vi "GE5565 DMA Read Interrupt (U64) Cluster.vi"(6 "timeout (1000 ms)":u32=1000, 8 "error in (no error)":errorcluster, 10 "RM offset (0)":u32, 11 "VMIC reference in":T1) -> (0 "error out":errorcluster, 2 "buffer":dbl[](array[numeric]), 3 "VMIC reference out":T1)   [LabVIEW 2020, in "RefMem DMA Engine.lvlib"]
uses:
  RefMem DMA Engine.lvlib
  <vilib>/Instr/_visa.llb/Select Event Type.ctl
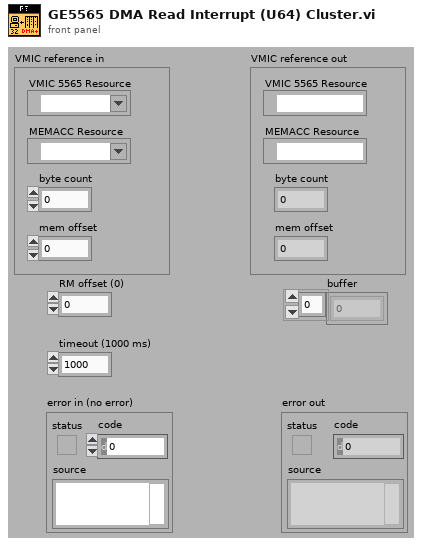
[diagram p1: front panel]
types:
  T1 = cluster{"VMIC 5565 Resource":refnum<visa-resource-name>, "MEMACC Resource":refnum<visa-resource-name>, "byte count":u32, "mem offset":u32}
  T2 = enum16{"big-endian, network order", "native, host order", "little-endian"}
  T3 = typedef "Select Event Type.ctl" = u32
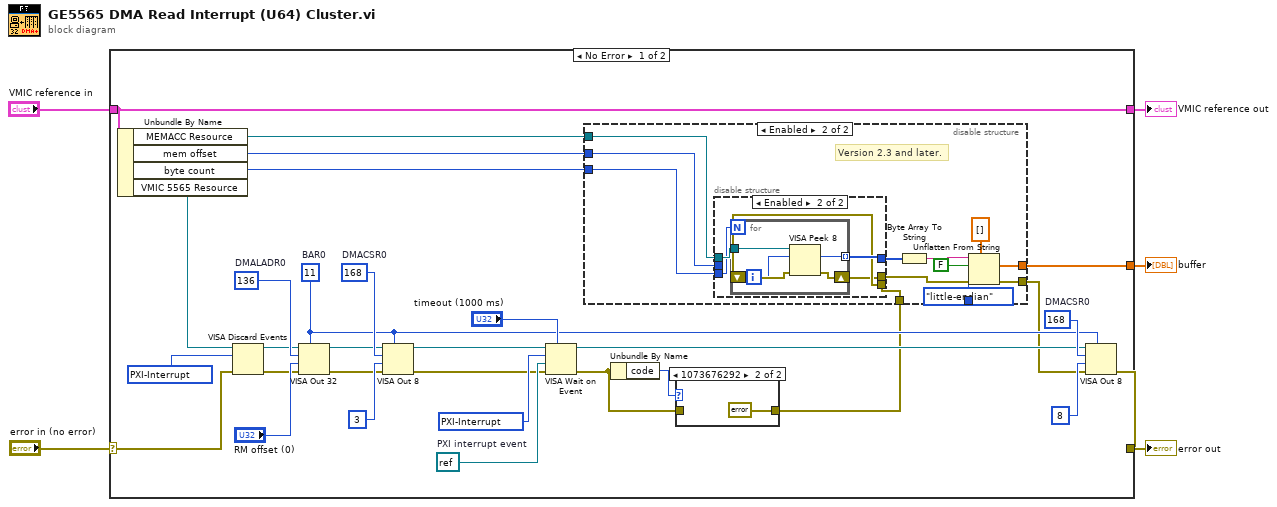
[diagram p0: block diagram]
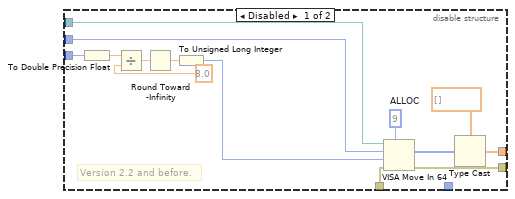
[diagram p2: hidden frame]
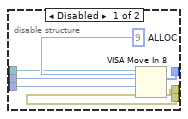
[diagram p3: hidden frame]
diagram:
  n1 = case shown="No Error" "error in (no error)" {
    selector: "error in (no error)" -> [w26 w82]
    tunnel: "VMIC reference in" -> [w21 w83]
    tunnel: [w21 w83] -> w2
    tunnel: [w11 w82] -> w4
    tunnel: [w10 _] -> w1
    frame No Error {
      w13 = u16 11  # BAR0
      w28 = refnum<visa-resource-name> refnum  # PXI interrupt event
      w16 = u32 168  # DMACSR0
      w23 = T3 1073684514 items=["ServiceRequest"=1073684491, "Trigger"=3221168138, "Clear"=1073684493, "VXI-Signal"=1073684512, "VXI/VME-Interrupt"=3221168161, "VXI/VME-Sysfail"=1073684509, "VXI/VME-Sysreset"=1073684510, "GPIB-CIC"=1073684498, "GPIB-Talk"=1073684499, "GPIB-Listen"=1073684500, "PXI-Interrupt"=1073684514, "AllEnabled"=1073709055] ("Event Type")
      w29 = T3 1073684514 items=["ServiceRequest"=1073684491, "Trigger"=3221168138, "Clear"=1073684493, "VXI-Signal"=1073684512, "VXI/VME-Interrupt"=3221168161, "VXI/VME-Sysfail"=1073684509, "VXI/VME-Sysreset"=1073684510, "GPIB-CIC"=1073684498, "GPIB-Talk"=1073684499, "GPIB-Listen"=1073684500, "PXI-Interrupt"=1073684514, "AllEnabled"=1073709055] ("Event Type")
      w35 = u32 168  # DMACSR0
      w36 = u32 136  # DMALADR0
      n2 = Unbundle By Name(w21) -> ("MEMACC Resource"=w18:refnum<visa-resource-name>, "mem offset"=w19:u32, "byte count"=w20:u32, "VMIC 5565 Resource"=w22:refnum<visa-resource-name>)
      n3 = VISA Discard Events(8:w26, 10:w23, 11:w22) -> (0:w24:errorcluster, 3:w25:refnum<visa-resource-name>)  [unwired: 1 in]
      n4 = VISA Out 32(7:w13, 8:w24, 9:"RM offset (0)", 10:w36, 11:w25) -> (0:w32:errorcluster, 3:w33:refnum<visa-resource-name>)
      n5 = VISA Out 8(7:w13, 8:w32, 9:u8 3 ("value (0)"), 10:w35, 11:w33) -> (0:w17:errorcluster, 3:w27:refnum<visa-resource-name>)
      n6 = VISA Wait on Event(7:"timeout (1000 ms)", 8:w17, 9:w28, 10:w29, 11:w27) -> (0:w9:errorcluster, 3:w14:refnum<visa-resource-name>)  [unwired: 2 out]
      n7 = Unbundle By Name(w9) -> ("code"=w7:i32)
      n8 = case shown="1073676292" w7 {
        tunnel: [w80 errorcluster {"status"=FALSE, "code"=0, "source"=""} ("error out")] -> w8
        tunnel: w9 -> [w80 _]
        frame 0, Default {
        }
        frame 1073676292 {
        }
      }
      n9 = disable-structure shown="Enabled" {
        disable-tunnel: w20 -> [w44 w52]
        disable-tunnel: w19 -> [w43 w53]
        disable-tunnel: w18 -> [w42 w54]
        disable-tunnel: [w41 w56] -> w12
        disable-tunnel: [w38 w57] -> w10
        disable-tunnel: w8 -> [w37 w55]
        disable-tunnel: T2."little-endian" ("byte order (0:big-endian, network order)") -> [_ w51]
        frame Disabled {
          w50 = u16 9  # ALLOC
          # "Version 2.2 and before."
          n10 = To Double Precision Float(number=w44) -> (double precision float=w49:dbl)
          n11 = Divide(x=w49, y=8.0) -> (x/y=w47:dbl)
          n12 = Round Toward -Infinity(1:w47) -> (0:w46:dbl)
          n13 = To Unsigned Long Integer(number=w46) -> (unsigned 32bit integer=w45:u32)
          n14 = VISA Move In 64(7:w50, 8:w37, 9:w45, 10:w43, 11:w42) -> (0:w41:errorcluster, 2:w40:u64[])  [unwired: 1 out]
          n15 = Type Cast(type=dbl[] [] ("buffer"), x=w40) -> (*(type *) &x=w38:dbl[])
        }
        frame Enabled {
          # "Version 2.3 and later."
          n16 = disable-structure shown="Enabled" {
            disable-tunnel: [w69 w74] -> w62
            disable-tunnel: [w68 w72] -> w61
            disable-tunnel: w55 -> [w67 w73]
            disable-tunnel: w54 -> [w65 w71]
            disable-tunnel: w53 -> [w64 _]
            disable-tunnel: w52 -> [w63 w70]
            frame Disabled {
              w66 = u16 9  # ALLOC
              n17 = VISA Move In 8(7:w66, 8:w67, 9:w63, 10:w64, 11:w65) -> (0:w68:errorcluster, 2:w69:u8[])  [unwired: 1 out]
            }
            frame Enabled {
              n18 = for {
                N: w70 -> [_]
                tunnel: [w79] -> w74 mode=indexing
                shift-right: [w77] -> w72
                shift-left: w73 -> [w78]
                tunnel: w71 -> [w76]
                i -> [w75]
                n19 = VISA Peek 8(8:w78, 10:w75, 11:w76) -> (0:w77:errorcluster, 2:w79:u8)  [unwired: 1 out]
              }
            }
          }
          n20 = Byte Array To String(unsigned byte array=w62) -> (string=w60:string)
          n21 = Unflatten From String(type=dbl[] [], binary string=w60, data includes array or string size? (T)=FALSE, byte order (0:big-endian, network order)=w51, error in (no error)=w61) -> (value=w57:dbl[], error out=w56:errorcluster)  [unwired: 1 out]
        }
      }
      n22 = VISA Out 8(7:w13, 8:w12, 9:u8 8 ("value (0)"), 10:w16, 11:w14) -> (0:w11:errorcluster)  [unwired: 1 out]
    }
    frame Error {
    }
  }
  "error out" <- w4
  "VMIC reference out" <- w2
  "buffer" <- w1
